vi "fire global stop.vi"(11 "Template in":refnum<class "Template.lvclass">) -> ()   [LabVIEW 2020, in "Template.lvlib" / "Template.lvclass"]
uses:
  Template.lvclass
  Template.lvclass/Template.ctl
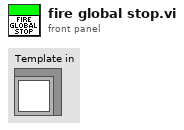
[diagram p1: front panel]
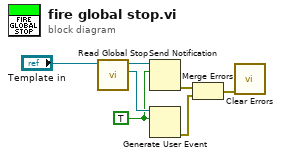
[diagram p0: block diagram]
diagram:
  w4 = TRUE ("notification")
  n1 = call "Read Global Stop.vi"("Template in"="Template in") -> ("Global Stop Event"=w5:refnum<user-event>, "Global Stop Notifier"=w6:refnum<notifier>)  [unwired: 9 in]
  n2 = Send Notification(notification=w4, notifier=w6) -> (error out=w3:errorcluster)  [unwired: 1 in, 1 out]
  n3 = Generate User Event(user event=w5, event data cluster=w4) -> (error out=w2:errorcluster)  [unwired: 2 in, 1 out]
  n4 = Merge Errors(w3, w2) -> (w1:errorcluster)
  n5 = call <vilib>:"Clear Errors.vi"("error in (no error)"=w1) -> ()  [unwired: 5 in, 2 out]
